vi "bronkhorst_Z.vi"(6 "T":u32[](array[numeric])=[1000, 10000, 300, 180000, 300, 5000, 180000, 3000], 7 "Alarm":bool[](array[boolean])=[FALSE, FALSE], 9 "ZB":bool, 10 "XB24":bool, 11 "Z_in":T5={"Z_HSw"=1, "Z_HSetState"=enum."on", "Z_ASetState"=enum."on", "Z_DSetState"=enum."on"}) -> (1 "ALR_ON":bool[](array[boolean]), 3 "Z":T1={"Z_Source"=enum."local disabled", "Z_SetState"=enum."on", "Z_State"=enum."alarm", "Z_State_T"=0, "ALR  L1"=FALSE, "ALR  L2"=FALSE, "HH_run"=0}, 4 "Z_State_next":u32)   [LabVIEW 2019]
uses:
  ctl/Z_State.ctl
  ctl/Z.ctl
  Heating/ctl/Y_source.ctl
  Heating/ctl/Z_State.ctl
  Sequence/State1.vi
  Trigers/RS.vi
  Timer Delay/Timer.vi
  Heating/Heating.lvlib
  control.lvlib
panel:
  # "Alarm_L1"
  # "Alarm_L2"
  # "XB24 local hand on"
  # "heating end"
  # "TsStop"
  # "T_check"
  # "T_start_delay"
  # "T_heat_start"
  # "T_stop_delay"
  # "T_set_min"
  # "T_heat_stop"
  # "T_restart_delay"
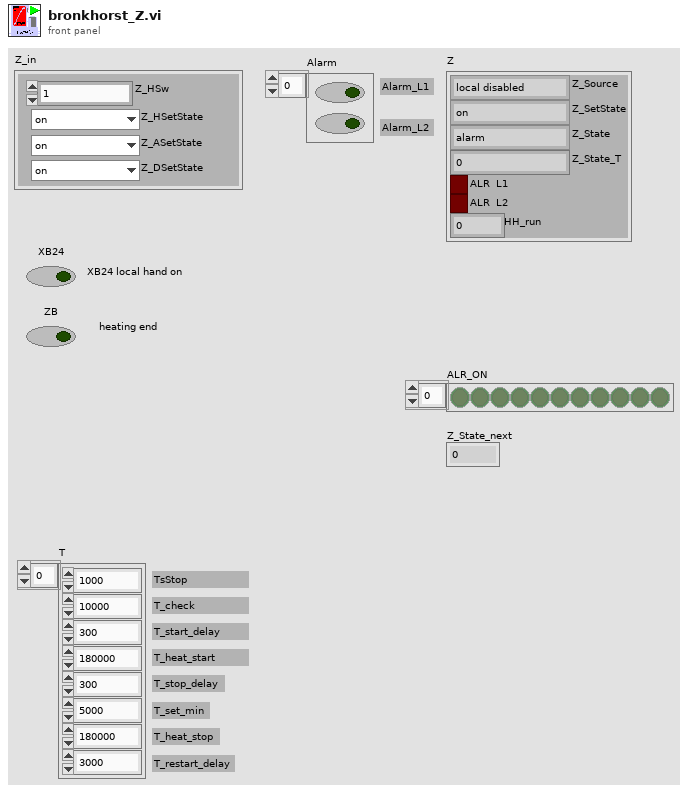
[diagram p1: front panel]
types:
  T1 = typedef "Z.ctl" = cluster{"Z_Source":T2, "Z_SetState":T3, "Z_State":T3, "Z_State_T":u32, "ALR  L1":bool, "ALR  L2":bool, "HH_run":i32}
  T2 = typedef "Heating.lvlib/Y_source.ctl" = enum8{"initialize", "local disabled", "local hand", "hand", "auto", "dist"}
  T3 = typedef "Heating.lvlib/Z_State.ctl" = enum8{"initialization", "alarm", "disabled", "not ready", "stop ready", "reserv", "switched off", "reserv2", "switched on", "check", "on min", "decrease out", "on", "increase out", "on max"}
  T4 = typedef "control.lvlib/Z_State.ctl" = enum8{"initialization", "alarm", "disabled", "not ready", "stop ready", "reserv", "switched off", "reserv2", "switched on", "check", "on min", "decrease out", "on", "increase out", "on max"}
  T5 = cluster{"Z_HSw":u32, "Z_HSetState":T4, "Z_ASetState":T4, "Z_DSetState":T4}
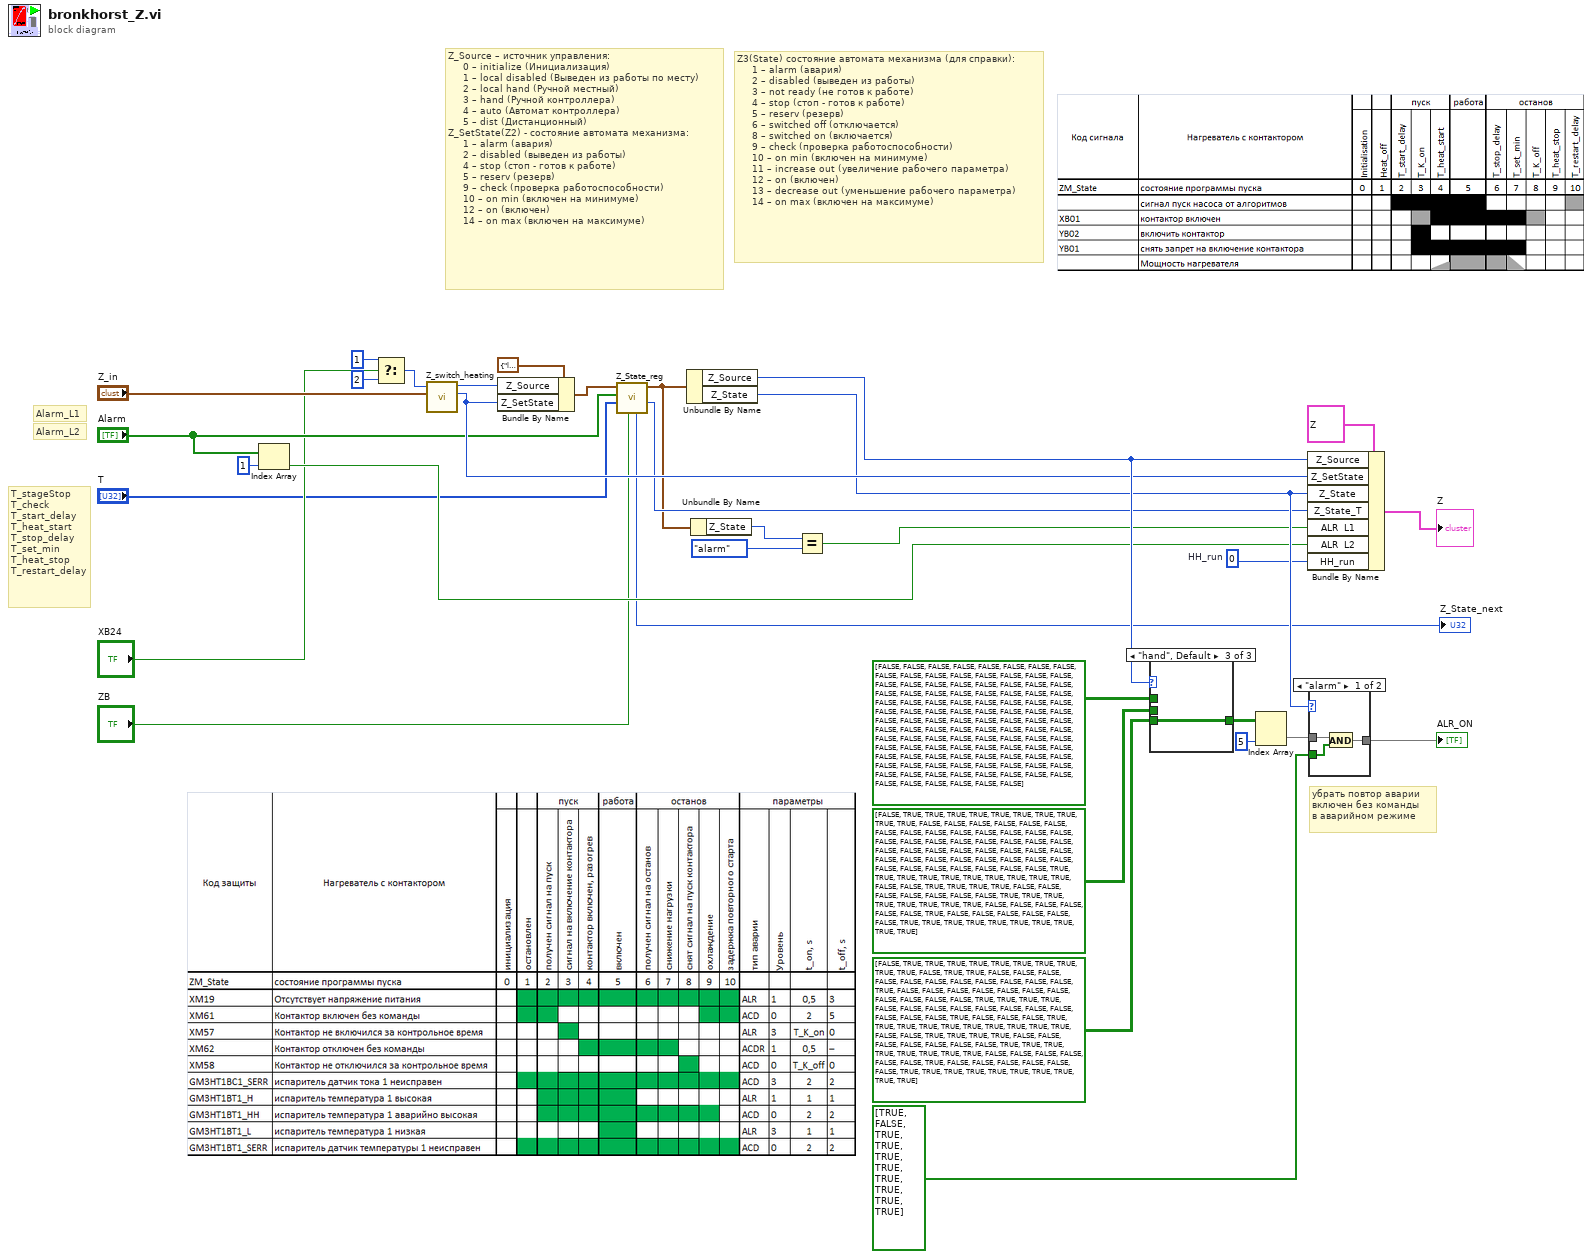
[diagram p0: block diagram]
diagram:
  w13 = 0  # HH_run
  # "Alarm_L2"
  # "Alarm_L1"
  # "T_stageStop\nT_check\nT_start_delay\nT_heat_start\nT_stop_delay\nT_set_min\nT_heat_stop\nT_restart_delay"
  # "убрать повтор аварии\nвключен без команды\nв аварийном режиме"
  # "Z_Source – источник управления:\n     0 – initialize (Инициализация)\n     1 – local disabled (Выведен из работы по месту)\n     2 – local hand (Ручной местный)\n     3 – hand (Ручной контроллера)\n     4 – auto (Автомат контроллера)\n     5 – dist (Дистанционный)\nZ_SetState(Z2) - состояние автомата механизма:\n     1 – alarm (авария)\n     2 – disabled (выведен из работы)\n     4 – stop (стоп - готов к работе)\n     5 – reserv (резерв)\n     9 – check (проверка работоспособности)\n     10 – on min (включен на минимуме)\n     12 – on (включен)\n     14 – on max (включен на максимуме)"
  # "Z3(State) состояние автомата механизма (для справки):\n     1 – alarm (авария)\n     2 – disabled (выведен из работы)\n     3 – not ready (не готов к работе)\n     4 – stop (стоп - готов к работе)\n     5 – reserv (резерв)\n     6 – switched off (отключается)\n     8 – switched on (включается)\n     9 – check (проверка работоспособности)\n     10 – on min (включен на минимуме)\n     11 – increase out (увеличение рабочего параметра)\n     12 – on (включен)\n     13 – decrease out (уменьшение рабочего параметра)\n     14 – on max (включен на максимуме)"
  n1 = Index Array(array="Alarm", index=1) -> (element=w8:bool)
  n2 = Select(t=u32 1, s="XB24", f=u32 2) -> (s? t:f=w27:u32)
  n3 = call "Z_switch_heating.vi"("Z"="Z_in", "Z_LSw"=w27) -> ("Z_SetState"=w18:T3, "Z_Source"=w25:T2)  [unwired: 8 in]
  n4 = Bundle By Name(cluster=cluster{"Z_Source":T2, "Z_SetState":T3} {"Z_Source"=enum."local disabled", "Z_SetState"=enum."alarm"} ("Z_In"), "Z_Source"=w25, "Z_SetState"=w18) -> (w24:cluster{"Z_Source":T2, "Z_SetState":T3})
  n5 = call "Z_State_reg.vi"("ZB"="ZB", "Time"="T", "Alarm"="Alarm", "Z_In"=w24) -> ("t"=w16:u32, "Z_Out"=w6:cluster{"Z_Source":T2, "Z_State":T3}, "N next"=→"Z_State_next":u32)  [unwired: 5 in]
  n6 = Unbundle By Name(w6) -> ("Z_Source"=w19:T2, "Z_State"=w17:T3)
  n7 = Unbundle By Name(w6) -> ("Z_State"=w11:T3)
  n8 = Equal?(x=w11, y=Z_State."alarm") -> (x = y?=w10:bool)
  n9 = case shown="\"hand\", Default" w19 {
    tunnel: bool[][] [[FALSE, FALSE, FALSE, FALSE, FALSE, FALSE, FALSE, FALSE, FALSE, FALSE, FALSE], [FALSE, FALSE, FALSE, FALSE, FALSE, FALSE, FALSE, FALSE, FALSE, FALSE, FALSE], [FALSE, FALSE, FALSE, FALSE, FALSE, FALSE, FALSE, FALSE, FALSE, FALSE, FALSE], [FALSE, FALSE, FALSE, FALSE, FALSE, FALSE, FALSE, FALSE, FALSE, FALSE, FALSE], [FALSE, FALSE, FALSE, FALSE, FALSE, FALSE, FALSE, FALSE, FALSE, FALSE, FALSE], [FALSE, FALSE, FALSE, FALSE, FALSE, FALSE, FALSE, FALSE, FALSE, FALSE, FALSE], [FALSE, FALSE, FALSE, FALSE, FALSE, FALSE, FALSE, FALSE, FALSE, FALSE, FALSE], [FALSE, FALSE, FALSE, FALSE, FALSE, FALSE, FALSE, FALSE, FALSE, FALSE, FALSE], [FALSE, FALSE, FALSE, FALSE, FALSE, FALSE, FALSE, FALSE, FALSE, FALSE, FALSE], [FALSE, FALSE, FALSE, FALSE, FALSE, FALSE, FALSE, FALSE, FALSE, FALSE, FALSE]] -> [w34 _ _]
    tunnel: bool[][] [[FALSE, TRUE, TRUE, TRUE, TRUE, TRUE, TRUE, TRUE, TRUE, TRUE, TRUE], [FALSE, FALSE, FALSE, FALSE, FALSE, FALSE, FALSE, FALSE, FALSE, FALSE, FALSE], [FALSE, FALSE, FALSE, FALSE, FALSE, FALSE, FALSE, FALSE, FALSE, FALSE, FALSE], [FALSE, FALSE, FALSE, FALSE, FALSE, FALSE, FALSE, FALSE, FALSE, FALSE, FALSE], [FALSE, FALSE, FALSE, FALSE, FALSE, FALSE, FALSE, FALSE, FALSE, FALSE, FALSE], [FALSE, TRUE, TRUE, TRUE, TRUE, TRUE, TRUE, TRUE, TRUE, TRUE, TRUE], [FALSE, FALSE, TRUE, TRUE, TRUE, TRUE, FALSE, FALSE, FALSE, FALSE, FALSE], [FALSE, FALSE, TRUE, TRUE, TRUE, TRUE, TRUE, TRUE, TRUE, TRUE, FALSE], [FALSE, FALSE, FALSE, FALSE, FALSE, TRUE, FALSE, FALSE, FALSE, FALSE, FALSE], [FALSE, TRUE, TRUE, TRUE, TRUE, TRUE, TRUE, TRUE, TRUE, TRUE, TRUE]] -> [_ w35 _]
    tunnel: bool[][] [[FALSE, TRUE, TRUE, TRUE, TRUE, TRUE, TRUE, TRUE, TRUE, TRUE, TRUE], [FALSE, TRUE, TRUE, FALSE, FALSE, FALSE, FALSE, FALSE, FALSE, FALSE, FALSE], [FALSE, FALSE, FALSE, TRUE, FALSE, FALSE, FALSE, FALSE, FALSE, FALSE, FALSE], [FALSE, FALSE, FALSE, FALSE, TRUE, TRUE, TRUE, TRUE, FALSE, FALSE, FALSE], [FALSE, FALSE, FALSE, FALSE, FALSE, FALSE, FALSE, FALSE, TRUE, FALSE, FALSE], [FALSE, TRUE, TRUE, TRUE, TRUE, TRUE, TRUE, TRUE, TRUE, TRUE, TRUE], [FALSE, FALSE, TRUE, TRUE, TRUE, TRUE, FALSE, FALSE, FALSE, FALSE, FALSE], [FALSE, FALSE, TRUE, TRUE, TRUE, TRUE, TRUE, TRUE, TRUE, TRUE, FALSE], [FALSE, FALSE, FALSE, FALSE, FALSE, TRUE, FALSE, FALSE, FALSE, FALSE, FALSE], [FALSE, TRUE, TRUE, TRUE, TRUE, TRUE, TRUE, TRUE, TRUE, TRUE, TRUE]] -> [_ _ w36]
    tunnel: [w34 w35 w36] -> w31
    frame "local disabled" {
    }
    frame "local hand" {
    }
    frame "hand", Default {
    }
  }
  n10 = Index Array(array=w31, index (col)=5 ("disabled index (col)")) -> (element=w30:bool[])  [unwired: 1 in]
  n11 = Bundle By Name(cluster=T1 {"Z_Source"=enum."local disabled", "Z_SetState"=enum."on", "Z_State"=enum."alarm", "Z_State_T"=0, "ALR  L1"=FALSE, "ALR  L2"=FALSE, "HH_run"=0} ("Z"), "Z_Source"=w19, "Z_SetState"=w18, "Z_State"=w17, "Z_State_T"=w16, "ALR  L1"=w10, "ALR  L2"=w8, "HH_run"=w13) -> (→"Z":T1)
  n12 = case shown="\"alarm\"" w17 {
    tunnel: bool[] [TRUE, FALSE, TRUE, TRUE, TRUE, TRUE, TRUE, TRUE, TRUE, TRUE] -> [w38 _]
    tunnel: w30 -> [w39 w40]
    tunnel: [w37 w40] -> w29
    frame "alarm" {
      n13 = And(x=w39, y=w38) -> (x .and. y?=w37:bool[])
    }
    frame "disabled", Default {
    }
  }
  "ALR_ON" <- w29
